vi "Unit Test.vi"() -> ()   [LabVIEW 2015, in "Peltier.lvclass"]
uses:
  Peltier.lvclass
panel:
  out "error out":errorcluster
  out "Side 2 Current":dbl
  out "Side 1 Current":dbl
  out "Side 2 Voltage":dbl
  out "Side 1 Voltage":dbl
  out "Serial Number":string
  out "Hardware Version":string
  out "Firmware Version":string
  out "Ready?":bool
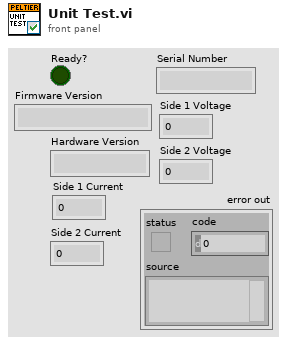
[diagram p1: front panel]
types:
  T1 = typedef "Peltier.lvclass/Session Handle.ctl" = refnum<data-value>
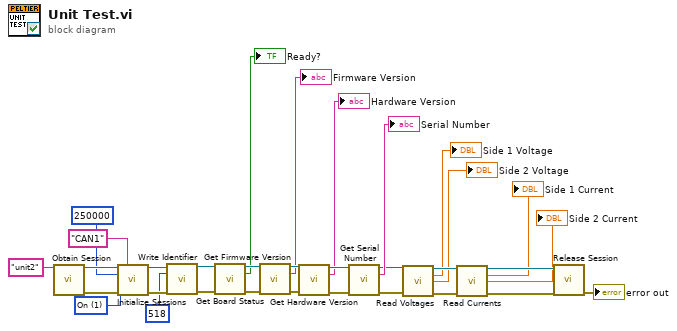
[diagram p0: block diagram]
diagram:
  w28 = u32 1 items=["Off", "On"] ("Termination")
  n1 = call "Obtain Session.vi"("Session  Name ()"="unit2") -> ("Session Handle"=w31:T1, "error out"=w30:errorcluster)  [unwired: 13 in]
  n2 = call "Initialize Sessions.vi"("Session Handle"=w31, "CAN Interface"="CAN1", "Baud Rate"=u32 250000, "Termination"=w28, "error in (no error)"=w30) -> ("Session Handle Out"=w27:T1, "error out"=w26:errorcluster)  [unwired: 9 in]
  n3 = call "Write Identifier.vi"("Session Handle In"=w27, "identifier"=u16 518, "error in (no error)"=w26) -> ("Session Handle Out"=w24:T1, "error out"=w23:errorcluster)  [unwired: 11 in]
  n4 = call "Get Board Status.vi"("Session Handle"=w24, "error in (no error)"=w23) -> ("Session Handle Out"=w22:T1, "Ready?"=→"Ready?":bool, "error out"=w17:errorcluster)  [unwired: 11 in]
  n5 = call "Get Firmware Version.vi"("Session Handle In"=w22, "error in (no error)"=w17) -> ("Session Handle Out"=w21:T1, "Firmware Version"=→"Firmware Version":string, "error out"=w16:errorcluster)  [unwired: 11 in]
  n6 = call "Get Hardware Version.vi"("Session Handle"=w21, "error in (no error)"=w16) -> ("Session Handle Out"=w20:T1, "Hardware Version"=→"Hardware Version":string, "error out"=w19:errorcluster)  [unwired: 11 in]
  n7 = call "Get Serial Number.vi"("Session Handle"=w20, "error in (no error)"=w19) -> ("Session Handle Out"=w12:T1, "Serial Number"=→"Serial Number":string, "error out"=w11:errorcluster)  [unwired: 11 in]
  n8 = call "Read Voltages.vi"("Session Handle"=w12, "error in (no error)"=w11) -> ("Session Handle Out"=w10:T1, "Side 1 Voltage"=→"Side 1 Voltage":dbl, "Side 2 Voltage"=→"Side 2 Voltage":dbl, "error out"=w9:errorcluster)  [unwired: 10 in]
  n9 = call "Read Currents.vi"("Session Handle"=w10, "error in (no error)"=w9) -> ("Session Handle Out"=w7:T1, "Side 1 Current"=→"Side 1 Current":dbl, "Side 2 Current"=→"Side 2 Current":dbl, "error out"=w8:errorcluster)  [unwired: 10 in]
  n10 = call "Release Session.vi"("Session Handle"=w7, "error in (no error)"=w8) -> ("error out"=→"error out":errorcluster)  [unwired: 13 in]
